vi "MoveF.vi"(0 "X":dbl, 5 "Y":dbl, 11 "error in (no error)":errorcluster) -> (15 "error out":errorcluster)   [LabVIEW 2019]
panel:
  in  "PID gains":T1={"proportional gain (Kc)"=0.3, "integral time (Ti, min)"=0.0, "derivative time (Td, min)"=0.0001}
  out "馬達電壓":dbl[][](graph)
  out "SPD":dbl[](graph)
  out "POS":dbl[](graph)
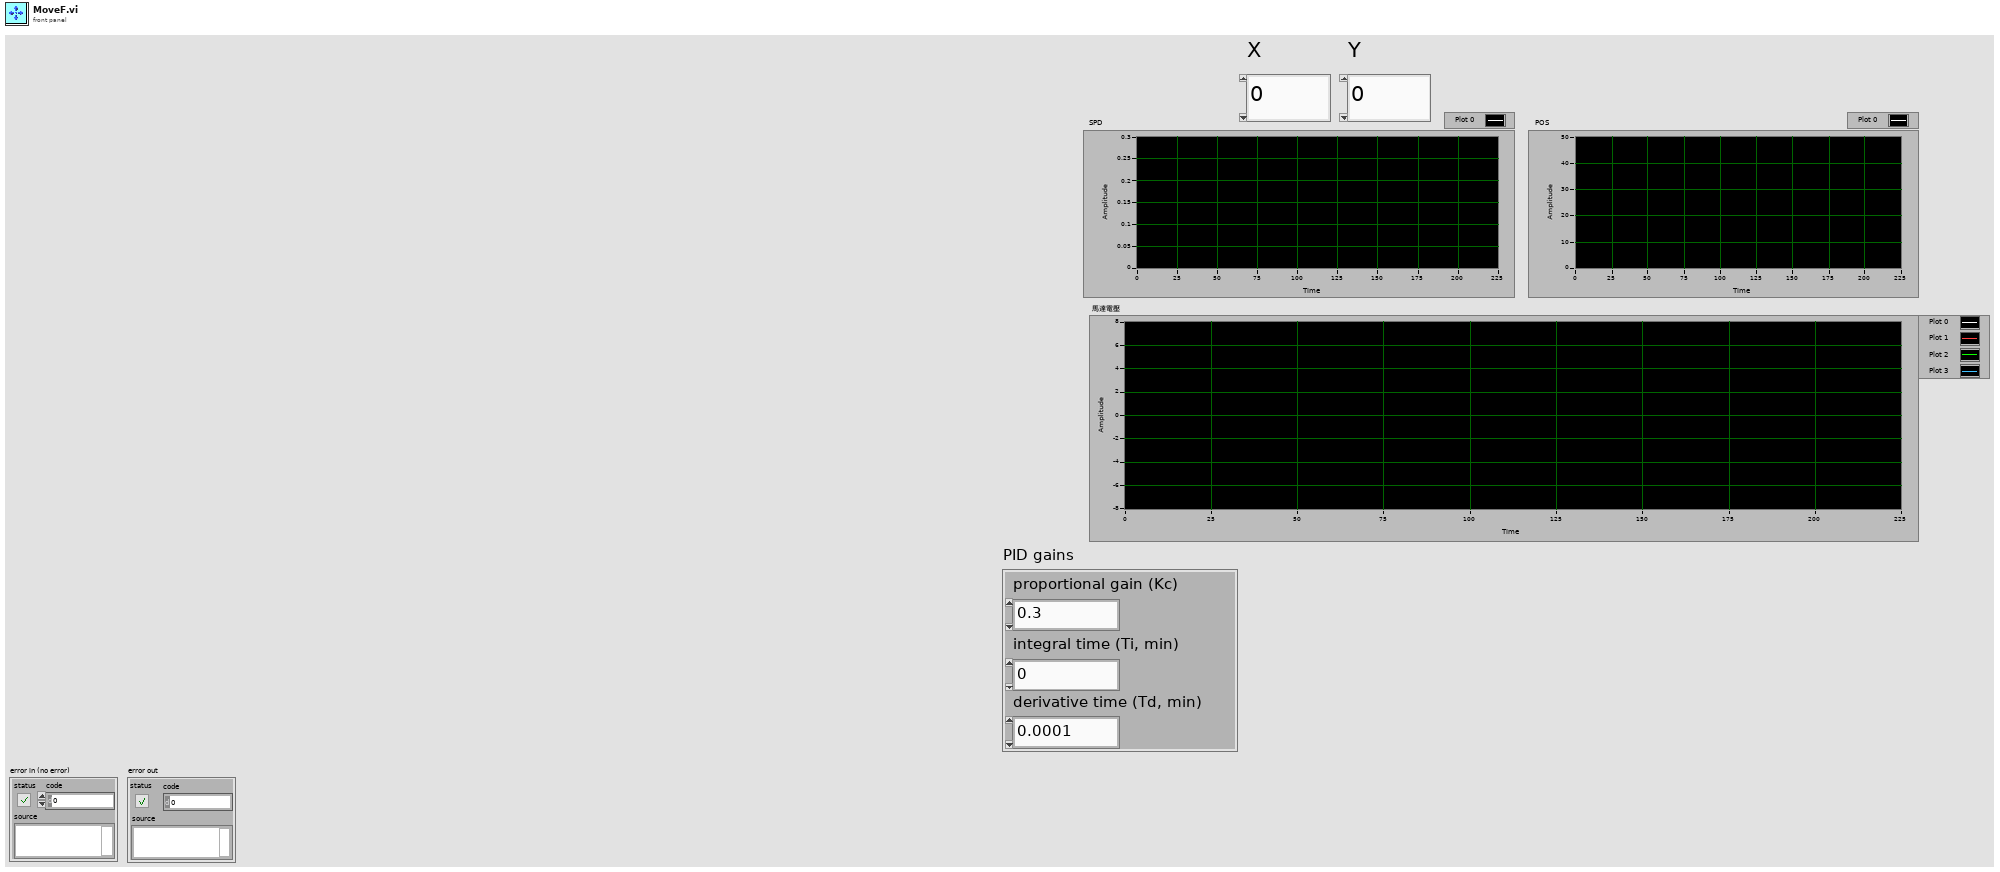
[diagram p1: front panel]
types:
  T1 = cluster{"proportional gain (Kc)":dbl, "integral time (Ti, min)":dbl, "derivative time (Td, min)":dbl}
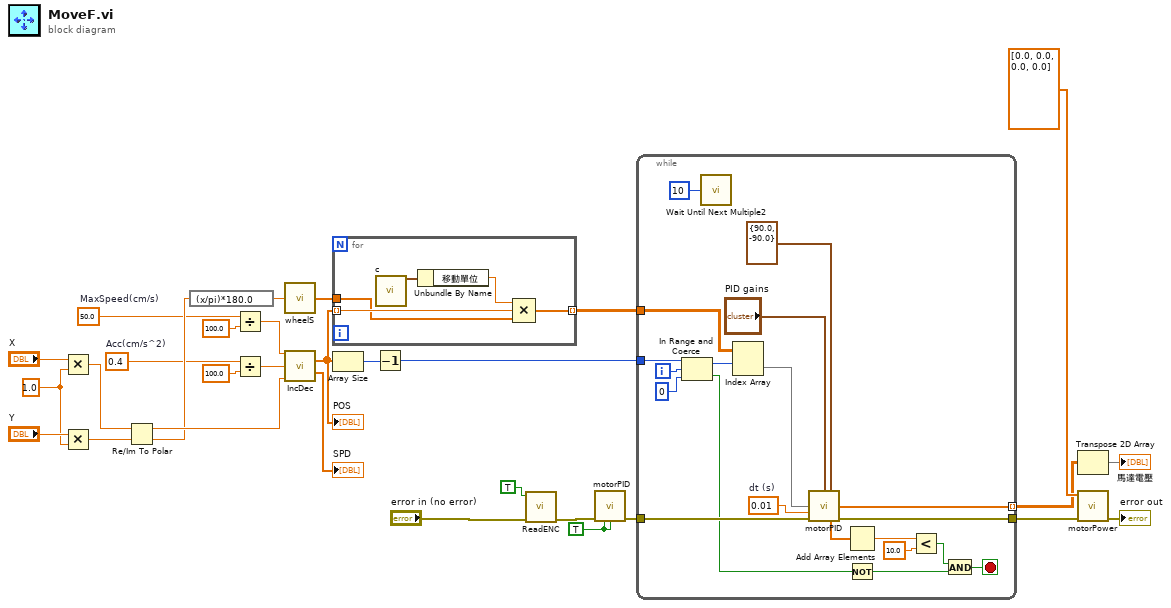
[diagram p0: block diagram]
diagram:
  w1 = 1.0 ("y")
  w14 = 0.4  # Acc(cm/s^2)
  w12 = 50.0  # MaxSpeed(cm/s)
  w26 = TRUE ("EncRst")
  n1 = Multiply(x="X", y=w1) -> (x*y=w4:dbl)
  n2 = Multiply(x="Y", y=w1) -> (x*y=w3:dbl)
  n3 = Re/Im To Polar(2:w3, 3:w4) -> (0:w16:dbl, 1:w19:dbl)
  n4 = expression code="(x/pi)*180.0" ("radians to degrees")(w16) -> (w20:dbl)
  n5 = Divide(x=w12, y=100.0) -> (x/y=w17:dbl)
  n6 = Divide(x=w14, y=100.0) -> (x/y=w18:dbl)
  n7 = call "wheelS.vi"("方向"=w20) -> ("輪速比"=w8:dbl[])  [unwired: 14 in]
  n8 = call "IncDec.vi"("MaxSpeed"=w17, "Acc"=w18, "Target"=w19) -> ("Position"=w10:dbl[], "Speed"=→"SPD":dbl[])  [unwired: 11 in]
  "POS" <- w10
  n9 = for {
    tunnel: w10 -> [w35] mode=indexing
    tunnel: [w34] -> w6 mode=indexing
    tunnel: w8 -> [w31]
    n10 = call "c.vi"() -> ("移動單位"=w32:cluster{"移動單位":dbl, "自轉單位":dbl})  [unwired: 15 in]
    n11 = Unbundle By Name(w32) -> ("移動單位"=w33:dbl)
    n12 = Compound Arithmetic op=MULTIPLY(w33, w35, w31) -> (w34:dbl[])
  }
  n13 = Array Size(array=w10) -> (size(s)=w11:i32)
  n14 = Decrement(x=w11) -> (x-1=w7:i32)
  n15 = call "ReadENC.vi"("error in (no error)"="error in (no error)", "Reset"=TRUE) -> ("error out"=w24:errorcluster)  [unwired: 8 in, 1 out]
  n16 = call "motorPID.vi"("error in (no error)"=w24, "reinitialize? (F)"=w26, "EncRst"=w26) -> ("error out"=w25:errorcluster)  [unwired: 9 in, 3 out]
  n17 = while {
    tunnel: [w55] -> w21 mode=indexing
    tunnel: w25 -> [w53]
    tunnel: [w54] -> w29
    tunnel: w7 -> [w37]
    tunnel: w6 -> [w36]
    i -> [w40]
    stop <- w39 stop-if-true
    w43 = 0.01  # dt (s)
    n18 = In Range and Coerce(upper limit=w37, x=w40, lower limit=0) -> (coerced(x)=w49:i32, In Range?=w48:bool)
    n19 = call "Wait Until Next Multiple2"("Count(mSec)"=u32 10) -> ()  [unwired: 1 out]
    n20 = Index Array(array=w36, index (row)=w49) -> (element=w44:dbl[])  [unwired: 1 in]
    n21 = call "motorPID.vi"("PID gains"="PID gains", "output range"=cluster{"output high":dbl, "output low":dbl} {"output high"=90.0, "output low"=-90.0}, "目標"=w44, "dt (s)"=w43, "error in (no error)"=w53) -> ("power"=w55:dbl[], "差值"=w42:dbl[], "error out"=w54:errorcluster)  [unwired: 7 in, 1 out]
    n22 = Add Array Elements(numeric array=w42) -> (sum=w52:dbl)
    n23 = Not(x=w48) -> (.not. x?=w46:bool)
    n24 = Less?(x=w52, y=10.0) -> (x < y?=w47:bool)
    n25 = And(x=w47, y=w46) -> (x .and. y?=w39:bool)
  }
  n26 = Transpose 2D Array(2D array=w21) -> (transposed array=→"馬達電壓":dbl[][])
  n27 = call "motorPower.vi"("error in (no error)"=w29, "DC_Pwr"=dbl[] [0.0, 0.0, 0.0, 0.0]) -> ("error out"=→"error out":errorcluster)  [unwired: 9 in]
